vi "F Dwf Digital Out Counter Init Get.vi"(7 "pv":u32, 8 "error in (no error)":errorcluster, 9 "pfHigh":i32, 10 "idxChannel":i32, 11 "hdwf":i32) -> (0 "error out":errorcluster, 1 "pfHigh out":i32, 3 "function return":i32, 5 "pv out":u32)   [LabVIEW 2019, in "Olasdwf.lvlib"]
doc: "DWFAPI int FDwfDigitalOutCounterInitGet(HDWF hdwf, int idxChannel, int *pfHigh, unsigned int *pv);"
uses:
  Olasdwf.lvlib
  Windows/System32/dwf.dll
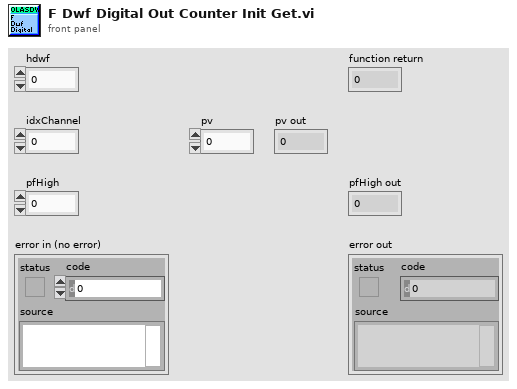
[diagram p1: front panel]
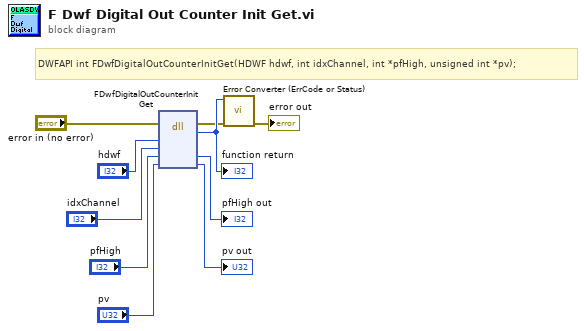
[diagram p0: block diagram]
diagram:
  # "DWFAPI int FDwfDigitalOutCounterInitGet(HDWF hdwf, int idxChannel, int *pfHigh, unsigned int *pv);"
  n1 = dll-call lib="C:/Windows/System32/dwf.*" fn="FDwfDigitalOutCounterInitGet"(error in="error in (no error)", "hdwf"="hdwf", "idxChannel"="idxChannel", "pfHigh"="pfHigh", "pv"="pv") -> (error out=w2:errorcluster, w10:i32, "pfHigh"=→"pfHigh out":i32, "pv"=→"pv out":u32)  [unwired: 4 in, 1 out]
  "function return" <- w10
  n2 = call "Error Converter (ErrCode or Status).vi"("error in (no error)"=w2, "error code"=w10) -> ("error out"=→"error out":errorcluster)  [unwired: 9 in]
